vi "Get Cells (1D Row Part String).vi"(6 "Column":i32, 8 "error in (no error)":errorcluster, 9 "Row":i32, 10 "Sheet Reference":refnum<k24>) -> (0 "error out":errorcluster, 2 "Sheet Reference out":refnum<k24>, 5 "Values":string[](array[string]))   [LabVIEW 2013]
doc: "Reads a row from the Sheet Reference. Row specifies which row to read from. Column specifies the starting column to read from (default of 0 for the full row)."
uses:
  C:/PhaeronGit/LVNPOI/Resources/NPOI 2.1.1 dotnet2/NPOI.dll
  Resources/NPOI 2.1.1 dotnet2/NPOI.dll
  <vilib>/ErrorRing/Error Ring.xnode
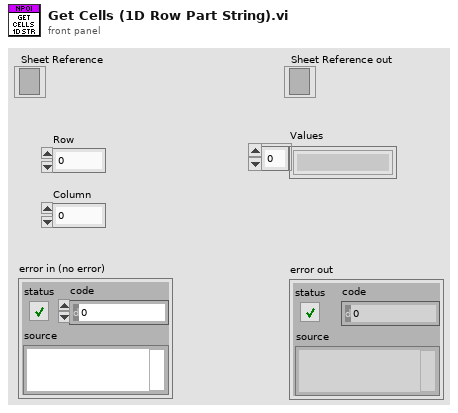
[diagram p1: front panel]
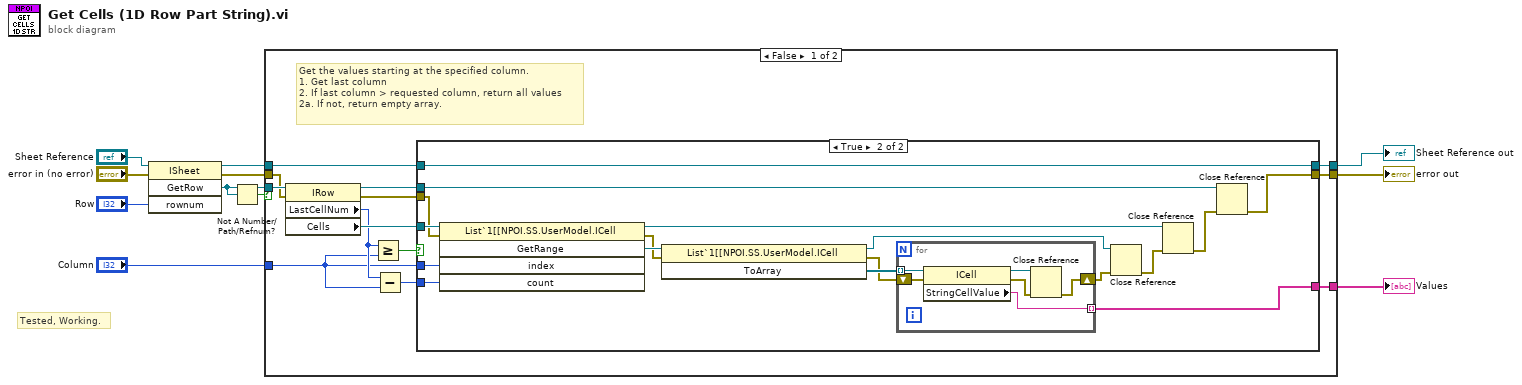
[diagram p0: block diagram]
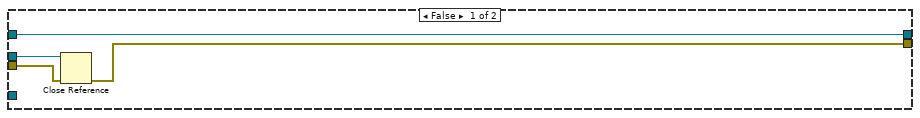
[diagram p2: hidden frame]
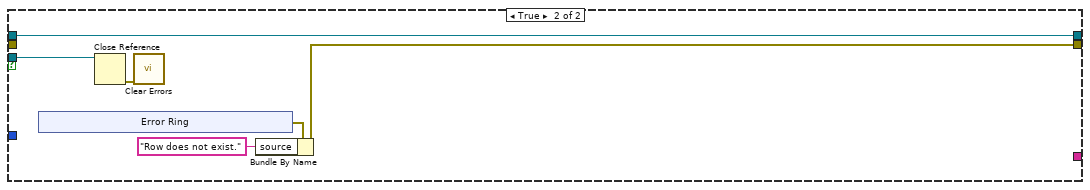
[diagram p3: hidden frame]
diagram:
  # "Tested, Working."
  n1 = invoke class="ISheet" method="GetRow"(reference="Sheet Reference", error in="error in (no error)", "rownum"="Row") -> (reference out=w8:refnum<k24>, error out=w9:errorcluster, "GetRow"=w11:refnum<k24>)  [unwired: 1 in, 1 out]
  n2 = Not A Number/Path/Refnum?(number/path/refnum=w11) -> (NaN/Path/Refnum?=w10:bool)
  n3 = case shown="False" w10 {
    tunnel: w8 -> [w16 w52]
    tunnel: w9 -> [w22 _]
    tunnel: [w17 w53] -> w2
    tunnel: [w15 w52] -> w4
    tunnel: w11 -> [w24 w54]
    tunnel: [w23 _] -> w3
    tunnel: "Column" -> [w13 _]
    frame False {
      # "Get the values starting at the specified column.\n1. Get last column\n2. If last column > requested column, return all values\n2a. If not, return empty array."
      n4 = property class="IRow"(reference=w24, error in=w22) -> (reference out=w19:refnum<k24>, error out=w18:errorcluster, "LastCellNum"=w14:i16, "Cells"=w21:refnum<k24>)
      n5 = Greater Or Equal?(x=w14, y=w13) -> (x >= y?=w20:bool)
      n6 = Subtract(x=w14, y=w13) -> (x-y=w12:i32)
      n7 = case shown="True" w20 {
        tunnel: [_ w44] -> w23
        tunnel: w21 -> [_ w42]
        tunnel: w19 -> [w28 w34]
        tunnel: w18 -> [w27 w40]
        tunnel: [w26 w32] -> w17
        tunnel: w16 -> [w25 w31]
        tunnel: [w25 w31] -> w15
        tunnel: w13 -> [_ w30]
        tunnel: w12 -> [_ w29]
        frame False {
          n8 = Close Reference(reference=w28, error in (no error)=w27) -> (error out=w26:errorcluster)
        }
        frame True {
          n9 = invoke class="List`1[[NPOI.SS.UserModel.ICell" method="GetRange"(reference=w42, error in=w40, "index"=w30, "count"=w29) -> (reference out=w36:refnum<k24>, error out=w39:errorcluster, "GetRange"=w43:refnum<k24>)  [unwired: 1 in, 2 out]
          n10 = invoke class="List`1[[NPOI.SS.UserModel.ICell" method="ToArray"(reference=w43, error in=w39) -> (reference out=w38:refnum<k24>, error out=w41:errorcluster, "ToArray"=w45:refnum<k24>[])  [unwired: 1 in]
          n11 = for {
            tunnel: w45 -> [w51] mode=indexing
            tunnel: [w50] -> w44 mode=indexing
            shift-right: [w47] -> w37
            shift-left: w41 -> [w46]
            n12 = property class="ICell"(reference=w51, error in=w46) -> (reference out=w48:refnum<k24>, error out=w49:errorcluster, "StringCellValue"=w50:string)
            n13 = Close Reference(reference=w48, error in (no error)=w49) -> (error out=w47:errorcluster)
          }
          n14 = Close Reference(reference=w38, error in (no error)=w37) -> (error out=w35:errorcluster)
          n15 = Close Reference(reference=w36, error in (no error)=w35) -> (error out=w33:errorcluster)
          n16 = Close Reference(reference=w34, error in (no error)=w33) -> (error out=w32:errorcluster)
        }
      }
    }
    frame True {
      n17 = xnode "Error Ring"() -> ("error out"=w56:errorcluster)
      n18 = Close Reference(reference=w54) -> (error out=w55:errorcluster)  [unwired: 1 in]
      n19 = call <vilib>:"Clear Errors.vi"("error in (no error)"=w55) -> ()  [unwired: 6 in, 1 out]
      n20 = Bundle By Name(cluster=w56, "source"="Row does not exist.") -> (w53:errorcluster)
    }
  }
  "Sheet Reference out" <- w4
  "error out" <- w2
  "Values" <- w3
